vi "Connect.vi"() -> (6 "TCP slave instance":refnum<class "Modbus Slave.lvclass">, 9 "error out":errorcluster)   [LabVIEW 2021]
uses:
  <vilib>/Modbus/slave/Modbus Slave.lvclass
  <vilib>/Modbus/slave/Create Slave Instance (TCP).vi
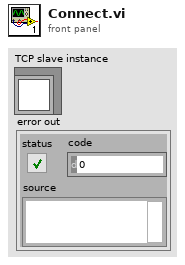
[diagram p1: front panel]
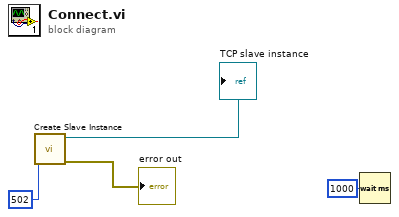
[diagram p0: block diagram]
diagram:
  n1 = call-poly <vilib>:"Create Slave Instance.vi"("port (502)"=u16 502) -> ("error out"=→"error out":errorcluster, "TCP slave instance"=→"TCP slave instance":refnum<class "Modbus Slave.lvclass">)  [unwired: 9 in]
  n2 = Wait (ms)(milliseconds to wait=u32 1000) -> ()  [unwired: 1 out]
